vi "Cartesian 2 Polar v1.vi"(0 "x":dbl, 1 "y":dbl, 2 "xcent":dbl, 3 "ycent":dbl, 4 "diam":dbl) -> (5 "r":dbl, 6 "t":dbl)   [LabVIEW 2014]
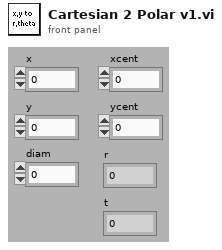
[diagram p1: front panel]
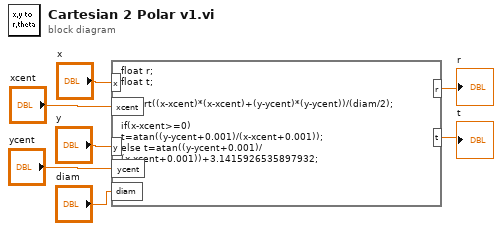
[diagram p0: block diagram]
diagram:
  n1 = formula code="float r;\nfloat t;\n\nr=sqrt((x-xcent)*(x-xcent)+(y-ycent)*(y-ycent))/(diam/2);\n\nif(x-xcent>=0)\nt=atan((y-ycent+0.001)/(x-xcent+0.001));\nelse t=atan((y-ycent+0.001)/(x-xcent+0.001))+3.1415926535897932;"("x"="x", "y"="y", "xcent"="xcent", "ycent"="ycent", "diam"="diam") -> ("r"=→"r":dbl, "t"=→"t":dbl)
